vi "CS_Gen_Save_Path.vi"(8 "error in (no error)":errorcluster) -> (0 "Error Out":errorcluster, 3 "Save path":path)   [LabVIEW 2018, in "Tracker.lvlib"]
uses:
  <vilib>/Utility/sysdir.llb/System Directory Type.ctl
  <userlib>/_OpenG.lib/md5/md5.llb/MD5 Message Digest (Hexadecimal String)__ogtk.vi
  Tracker.lvlib
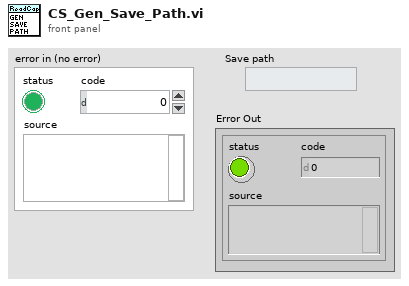
[diagram p1: front panel]
types:
  T1 = typedef "System Directory Type.ctl" = i32
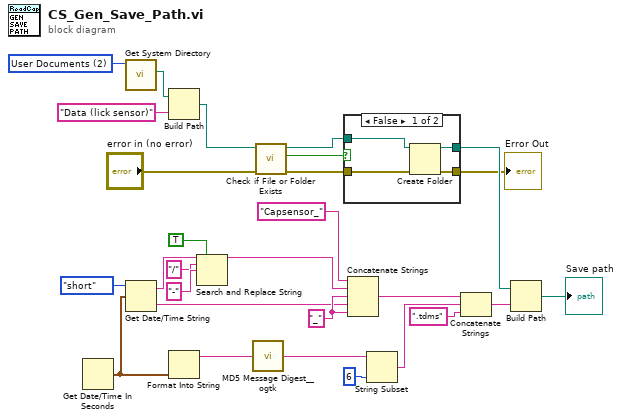
[diagram p0: block diagram]
diagram:
  w14 = "_" ("string")
  w2 = T1 2 items=["User Home"=0, "User Desktop"=1, "User Documents"=2, "User Application Data"=3, "User Preferences"=4, "User Temporary"=5, "Public Documents"=6, "Public Application Data"=7, "Public Preferences"=8, "Public Cache"=13, "System Core Libraries"=9, "System Installed Libraries"=10, "Application Files"=11, "Boot Volume Root"=12] ("system directory type")
  n1 = Get Date/Time In Seconds() -> (seconds since 1Jan1904=w23:timestamp)
  n2 = call <vilib>:"Get System Directory.vi"("system directory type"=w2) -> ("system directory"=w3:path)  [unwired: 10 in]
  n3 = Get Date/Time String(date format (0)=enum16{"short", "long", "abbreviated"}."short", seconds (now)=w23) -> (date string=w25:string, time string=w13:string)  [unwired: 1 in]
  n4 = Build Path(base path=w3, name or relative path="Data (lick sensor)") -> (appended path=w5:path)
  n5 = Format Into String(w23) -> (resulting string=w21:string)  [unwired: 3 in, 1 out]
  n6 = Search and Replace String(replace all?=TRUE ("replace all? (F)"), input string=w25, search string="/", replace string="-" ("replace string (\"\")")) -> (result string=w24:string)  [unwired: 4 in, 3 out]
  n7 = call-poly <userlib>:"MD5 Message Digest__ogtk.vi"("Message"=w21) -> ("MD5 Message Digest"=w20:string)
  n8 = call <vilib>:"Check if File or Folder Exists.vi"("error in (no error)"="error in (no error)", "path"=w5) -> ("error out"=w8:errorcluster, "file or folder exists?"=w6:bool, "dup path"=w7:path)  [unwired: 7 in]
  n9 = case shown="False" w6 {
    tunnel: w7 -> [w32 w34]
    tunnel: w8 -> [w31 w33]
    tunnel: [w30 w34] -> w10
    tunnel: [w29 w33] -> w1
    frame False {
      n10 = Create Folder(path (use dialog)=w32, error in=w31) -> (created path=w30:path, error out=w29:errorcluster)  [unwired: 1 in, 1 out]
    }
    frame True {
    }
  }
  "Error Out" <- w1
  n11 = Concatenate Strings("Capsensor_" ("string"), w24, w14, w13, w14) -> (w19:string)
  n12 = String Subset(string=w20, length (rest)=6 ("length (rest)")) -> (substring=w16:string)  [unwired: 1 in]
  n13 = Concatenate Strings(w19, w16, ".tdms" ("string")) -> (w17:string)
  n14 = Build Path(base path=w10, name or relative path=w17) -> (appended path=→"Save path":path)
